vi "Bound.vi"(11 "ComboBox in":refnum<vi>) -> (2 "Bound":T1, 3 "ComboBox out":refnum<vi>)   [LabVIEW 2017, in "UI_TimeSelector.xctl"]
uses:
  UI_TimeSelector.xctl
  <vilib>/Utility/miscctls.llb/LVRectTypeDef.ctl
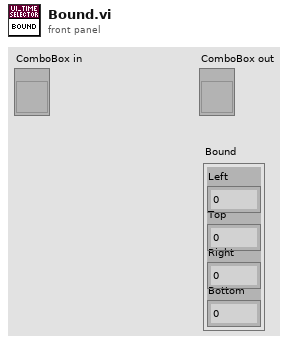
[diagram p1: front panel]
types:
  T1 = typedef "LVRectTypeDef.ctl" = cluster{"Left":i16, "Top":i16, "Right":i16, "Bottom":i16}
  T2 = typedef "LVPositionTypeDef.ctl" = cluster{"Left":i32, "Top":i32}
  T3 = typedef "LVBoundsTypeDef.ctl" = cluster{"Width":u32, "Height":u32}
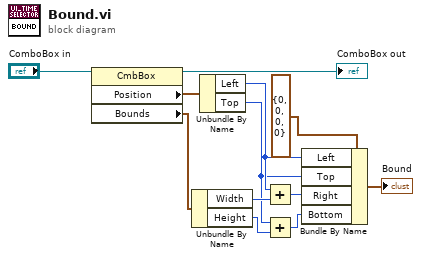
[diagram p0: block diagram]
diagram:
  n1 = property class="CmbBox"(reference="ComboBox in") -> (reference out=→"ComboBox out":refnum<vi>, "Position"=w10:T2, "Bounds"=w9:T3)  [unwired: 1 in, 1 out]
  n2 = Unbundle By Name(w9) -> ("Width"=w6:u32, "Height"=w3:u32)
  n3 = Unbundle By Name(w10) -> ("Left"=w5:i32, "Top"=w2:i32)
  n4 = Add(x=w5, y=w6) -> (x+y=w4:u32)
  n5 = Add(x=w2, y=w3) -> (x+y=w1:u32)
  n6 = Bundle By Name(cluster=T1 {"Left"=0, "Top"=0, "Right"=0, "Bottom"=0} ("Bound"), "Left"=w5, "Top"=w2, "Right"=w4, "Bottom"=w1) -> (→"Bound":T1)
